vi "Command (read & write) - DL.vi"(7 "timeout ms (100)":i32=100, 8 "error in (no error)":errorcluster, 9 "Parameter":i32, 10 "IP":string, 11 "connection ID in":refnum<k16>) -> (0 "error out":errorcluster, 2 "I32 Param out":i32, 3 "connection ID out":refnum<k16>)   [LabVIEW 2016, in "SMD-7615.lvlib" / "eSCL.lvlib"]
doc: "DL - Define Limits (StepSERVO and SV200 drives)\nCW and CCW end-of-travel limits are available on all drives and can be used to define the boundaries of\nacceptable motion in a motor/drive system. If one of these inputs is activated while defined as an end-of-travel limit, motor rotation will stop in that direction, and an alarm code will show at the drive’s status LEDs. When defining these inputs as end-of-travel limits, individual or both inputs can be defined as either active low, active high, or not used. See below for details.\n\nDL1: End-of-travel limit occurs when an input is closed (energized). Motion stops automatically at rate defined by AM command.\nDL2: End-of-travel limit occurs when an input is open (de-energized). Motion stops automatically at rated\ndefined by AM command.\nDL3: Inputs are not used as end-of-travel limit inputs and can be used as a general purpose inputs. In the case of ST-S and STM drives, DL will be automatically set to 3 if CM is set to 7, 11, 12, 13, 14, 15, 16, 17, or 18, or if JE is executed after the DL command is set.\nDL7: individually set end-of-travel in CW direction when CW Limit inputs is closed(energized).\nDL8: individually set end-of-travel in CW direction when CW Limit inputs is open (de-energized).\nDL9: individually set end-of-travel in CCW direction when CCW Limit inputs is closed(energized).\nDL10: individually set end-of-travel in CCW direction when CCW Limit inputs is open (de-energized).\nDL11~13, DL17~20: Swap the CW input and CCW input definition as above setting."
uses:
  eSCL.lvlib
  I32 Command and Param.ctl
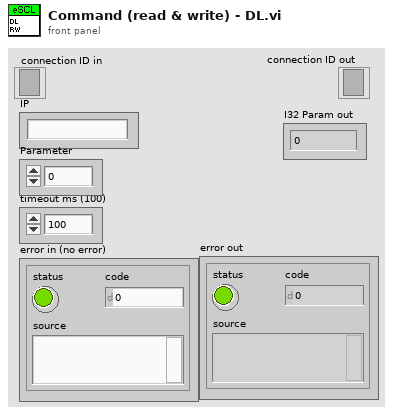
[diagram p1: front panel]
types:
  T1 = typedef "SMD-7615.lvlib/eSCL.lvlib/I32 Command and Param.ctl" = cluster{"Command":string, "I32 Parameler":i32, "I32 Parameler Default":i32, "I32 Parameler Coerece Upper":i32, "I32 Parameler Coerece Lower":i32}
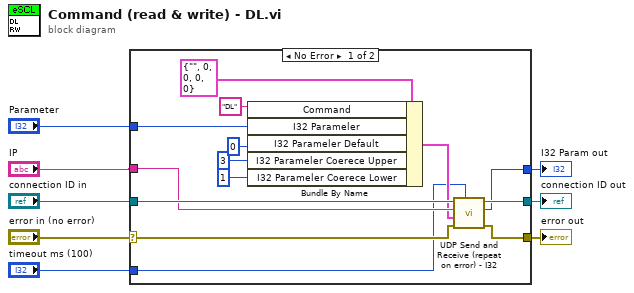
[diagram p0: block diagram]
diagram:
  n1 = case shown="No Error" "error in (no error)" {
    selector: "error in (no error)" -> [w16 w23]
    tunnel: "connection ID in" -> [w19 w24]
    tunnel: [w14 w24] -> w2
    tunnel: [w13 w23] -> w1
    tunnel: "IP" -> [w18 _]
    tunnel: "timeout ms (100)" -> [w15 _]
    tunnel: [w12 _] -> w3
    tunnel: "Parameter" -> [w9 _]
    frame No Error {
      n2 = Bundle By Name(cluster=T1 {"Command"="", "I32 Parameler"=0, "I32 Parameler Default"=0, "I32 Parameler Coerece Upper"=0, "I32 Parameler Coerece Lower"=0} ("I32 Command & Param"), "Command"="DL", "I32 Parameler"=w9, "I32 Parameler Default"=0 ("DBL Parameler Default"), "I32 Parameler Coerece Upper"=3 ("DBL Parameler Coerece Upper"), "I32 Parameler Coerece Lower"=1 ("DBL Parameler Coerece Lower")) -> (w17:T1)
      n3 = call "UDP Send and Receive (repeat on error) - I32.vi"("timeout ms (100)"=w15, "error in (no error)"=w16, "I32 Command & Param"=w17, "IP"=w18, "connection ID in"=w19) -> ("error out"=w13:errorcluster, "I32 Param out"=w12:i32, "connection ID out"=w14:refnum<k16>)  [unwired: 4 in]
    }
    frame Error {
    }
  }
  "connection ID out" <- w2
  "error out" <- w1
  "I32 Param out" <- w3
